vi "AKIP_measure_voltage_current.vi"(8 "error in (no error)":errorcluster, 11 "VISA Refnum in":refnum<visa-resource-name>="AKIP") -> (0 "error out":errorcluster, 1 "Current":dbl, 2 "Voltage":dbl, 3 "VISA Refnum out":refnum<visa-resource-name>)   [LabVIEW 2017]
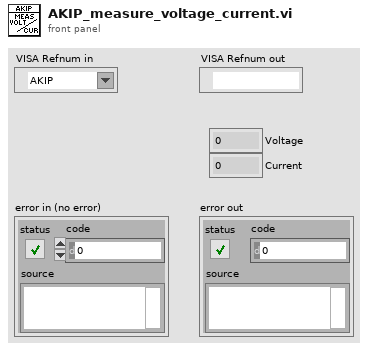
[diagram p1: front panel]
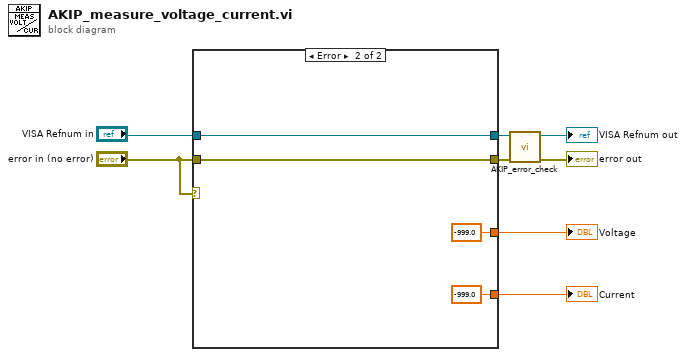
[diagram p0: block diagram]
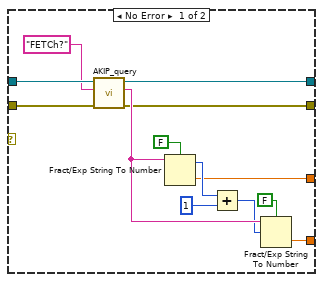
[diagram p2: hidden frame]
diagram:
  n1 = case shown="Error" "error in (no error)" {
    tunnel: "error in (no error)" -> [w15 w24]
    tunnel: "VISA Refnum in" -> [w14 w25]
    tunnel: [w12 w25] -> w7
    tunnel: [w11 w24] -> w6
    tunnel: [w10 -999.0] -> w3
    tunnel: [w9 -999.0] -> w2
    frame No Error {
      n2 = call "AKIP_query.vi"("error in (no error)"=w15, "write buffer"="FETCh?", "VISA Refnum in"=w14) -> ("error out"=w11:errorcluster, "read buffer"=w21:string, "VISA Refnum out"=w12:refnum<visa-resource-name>)  [unwired: 6 in]
      n3 = Fract/Exp String To Number(use system decimal point (T)=FALSE, string=w21) -> (offset past number=w19:i32, number=w10:dbl)  [unwired: 2 in]
      n4 = Add(x=w19, y=1) -> (x+y=w18:i32)
      n5 = Fract/Exp String To Number(use system decimal point (T)=FALSE, string=w21, offset=w18) -> (number=w9:dbl)  [unwired: 1 in, 1 out]
    }
    frame Error {
    }
  }
  "Voltage" <- w3
  "Current" <- w2
  n6 = call "AKIP_error_check.vi"("error in (no error)"=w6, "VISA Refnum in"=w7) -> ("error out"=→"error out":errorcluster, "VISA Refnum out"=→"VISA Refnum out":refnum<visa-resource-name>)  [unwired: 8 in]
